vi "Build Tree from Project.vi"(8 "error in":errorcluster, 11 "Project in":refnum<class "Project.lvclass">) -> (0 "error out":errorcluster, 2 "Tree Map Out":T1)   [LabVIEW 2019, in "Panther Dashboard.lvlib" / "Project.lvclass"]
uses:
  Project.lvclass
  <vilib>/National Instruments/Tree Map/Tree Map Data.ctl
  Panther Dashboard/Map Attribute--enum.ctl
  Project.lvclass/Project.ctl
  Library/Library.lvclass/Library.ctl
  VI/VI.lvclass/VI.ctl
  VI/Read VI Plain Name.vi
  VI/Read VI Path.vi
  Library/Read VIs MAP.vi
  Library/Read Library Name.vi
  Library/Read Library Path.vi
  Library/Read Type.vi
  Library/Read Dependency.vi
  Read Libraries.vi
  Read Project Name.vi
  Read Target Name.vi
  Read Project Path.vi
  Library/Library.lvclass
  VI/VI.lvclass
  <vilib>/National Instruments/Tree Map/Tree Map.lvlib
  Panther Dashboard/Panther Dashboard.lvlib
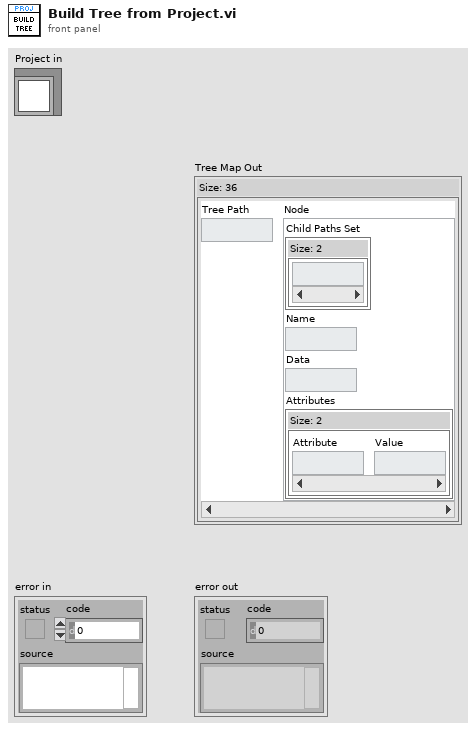
[diagram p1: front panel]
types:
  T1 = typedef "Tree Map.lvlib/Tree Map Data.ctl" = map{string, cluster{"Child Paths Set":set{string}, "Name":string, "Data":string, "Attributes":map{string, string}}}
  T2 = typedef "Panther Dashboard.lvlib/Map Attribute--enum.ctl" = enum16{"Path", "ModuleType", "Module Description", "Dependency?", "Target"}
  T3 = typedef "Panther Dashboard.lvlib/Library.lvclass/VI Type--enum.ctl" = enum16{"Requests", "Broadcasts", "Request and Wait for Reply", "Round Trips", "Public API VIs", "» Constant VIs", "» Error VIs"}
  T4 = typedef "Panther Dashboard.lvlib/Module type--enum.ctl" = enum16{"Singleton", "Cloneable"}
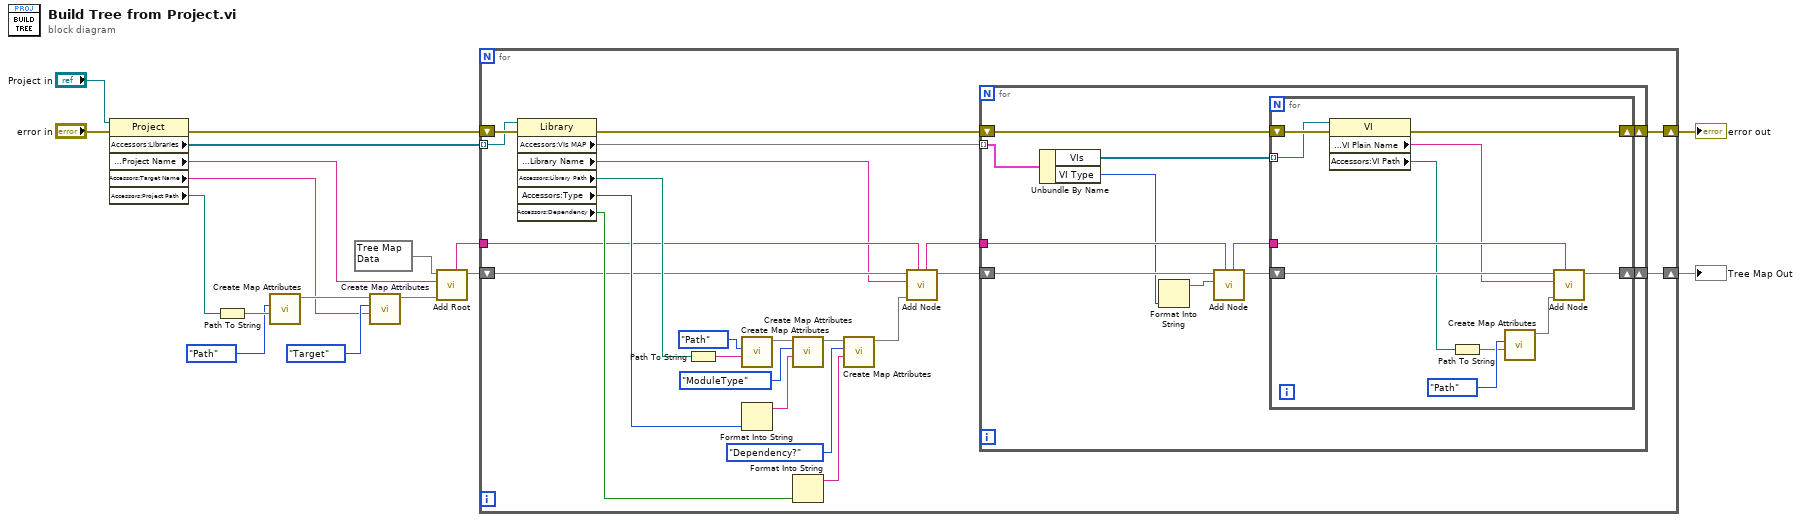
[diagram p0: block diagram]
diagram:
  n1 = property class="Project"(reference="Project in", error in="error in") -> (error out=w16:errorcluster, "Accessors:Libraries"=w6:refnum<class "Library.lvclass">[], "Accessors:Project Name"=w7:string, "Accessors:Target Name"=w2:string, "Accessors:Project Path"=w3:path)  [unwired: 1 out]
  n2 = Path To String(path=w3) -> (string=w13:string)
  n3 = call "Create Map Attributes.vi"("Attribute"=w13, "Map Attribute"=Map_Attribute--enum."Path") -> ("Root Attributes"=w12:map{string, string})  [unwired: 9 in]
  n4 = call "Create Map Attributes.vi"("Attribute"=w2, "Map Attribute"=Map_Attribute--enum."Target", "Root Attributes In"=w12) -> ("Root Attributes"=w11:map{string, string})  [unwired: 8 in]
  n5 = call <vilib>:"Add Root.vi"("Root Attributes"=w11, "New Root Name"=w7, "Tree Map In"=T1 {} ("Tree Map out")) -> ("Tree Map Out"=w5:T1, "Root Path"=w4:string)  [unwired: 7 in]
  n6 = for {
    shift-right: [w38] -> w15
    shift-left: w16 -> [w40]
    tunnel: w6 -> [w37] mode=indexing
    shift-right: [w20] -> w1
    shift-left: w5 -> [w25]
    tunnel: w4 -> [w23]
    n7 = property class="Library"(reference=w37, error in=w40) -> (error out=w39:errorcluster, "Accessors:VIs MAP"=w18:map{T3, refnum<class "VI.lvclass">[]}, "Accessors:Library Name"=w22:string, "Accessors:Library Path"=w35:path, "Accessors:Type"=w31:T4, "Accessors:Dependency"=w27:bool)  [unwired: 1 out]
    n8 = Path To String(path=w35) -> (string=w32:string)
    n9 = call "Create Map Attributes.vi"("Attribute"=w32, "Map Attribute"=Map_Attribute--enum."Path") -> ("Root Attributes"=w34:map{string, string})  [unwired: 9 in]
    n10 = Format Into String(w31) -> (resulting string=w28:string)  [unwired: 3 in, 1 out]
    n11 = call "Create Map Attributes.vi"("Attribute"=w28, "Map Attribute"=Map_Attribute--enum."ModuleType", "Root Attributes In"=w34) -> ("Root Attributes"=w30:map{string, string})  [unwired: 8 in]
    n12 = Format Into String(w27) -> (resulting string=w26:string)  [unwired: 3 in, 1 out]
    n13 = call "Create Map Attributes.vi"("Attribute"=w26, "Map Attribute"=Map_Attribute--enum."Dependency?", "Root Attributes In"=w30) -> ("Root Attributes"=w24:map{string, string})  [unwired: 8 in]
    n14 = call <vilib>:"Add Node.vi"("Parent Path"=w23, "Attributes"=w24, "New Node Name"=w22, "Tree Map In"=w25) -> ("Tree Map Out"=w21:T1, "New Node Path"=w19:string)  [unwired: 5 in, 1 out]
    n15 = for {
      shift-right: [w46] -> w20
      shift-left: w21 -> [w49]
      shift-right: [w50] -> w38
      shift-left: w39 -> [w51]
      tunnel: w19 -> [w47]
      tunnel: w18 -> [w43] mode=indexing
      n16 = Unbundle By Name(w43) -> ("VIs"=w41:refnum<class "VI.lvclass">[], "VI Type"=w42:T3)
      n17 = Format Into String(w42) -> (resulting string=w44:string)  [unwired: 3 in, 1 out]
      n18 = call <vilib>:"Add Node.vi"("Parent Path"=w47, "New Node Name"=w44, "Tree Map In"=w49) -> ("Tree Map Out"=w48:T1, "New Node Path"=w45:string)  [unwired: 6 in, 1 out]
      n19 = for {
        tunnel: w45 -> [w58]
        shift-right: [w61] -> w50
        shift-left: w51 -> [w62]
        shift-right: [w59] -> w46
        shift-left: w48 -> [w60]
        tunnel: w41 -> [w52] mode=indexing
        n20 = property class="VI"(reference=w52, error in=w62) -> (error out=w61:errorcluster, "Accessors:VI Plain Name"=w54:string, "Accessors:VI Path"=w53:path)  [unwired: 1 out]
        n21 = Path To String(path=w53) -> (string=w55:string)
        n22 = call "Create Map Attributes.vi"("Attribute"=w55, "Map Attribute"=Map_Attribute--enum."Path") -> ("Root Attributes"=w56:map{string, string})  [unwired: 9 in]
        n23 = call <vilib>:"Add Node.vi"("Parent Path"=w58, "Attributes"=w56, "New Node Name"=w54, "Tree Map In"=w60) -> ("Tree Map Out"=w59:T1)  [unwired: 5 in, 2 out]
      }
    }
  }
  "error out" <- w15
  "Tree Map Out" <- w1
